vi "Close.vi"(8 "error in (no error)":errorcluster, 11 "QueueReader in":refnum<class "MultiQueueReader.lvclass">) -> (0 "error out":errorcluster, 3 "QueueReader out":refnum<class "MultiQueueReader.lvclass">)   [LabVIEW 2013, in "MultiQueueReader.lvclass"]
doc: "Closes all open references and reserved resources for the reader"
uses:
  MultiQueueReader.lvclass
  BaseReader/BaseReader.lvclass
  MultiQueueReader.lvclass/MultiQueueReader.ctl
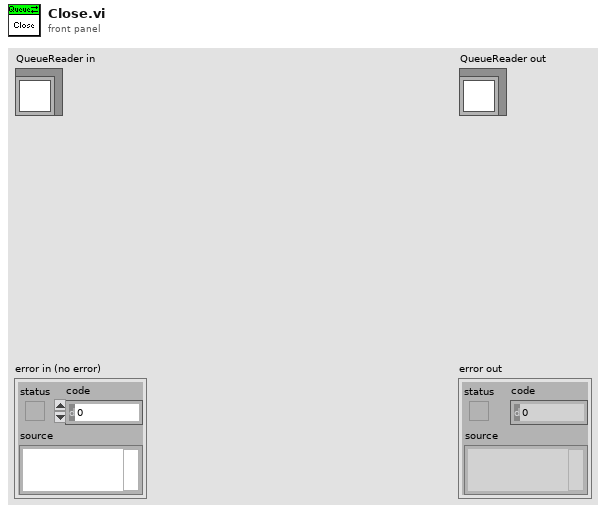
[diagram p1: front panel]
types:
  T1 = typedef "response queue.ctl" = refnum<queue>
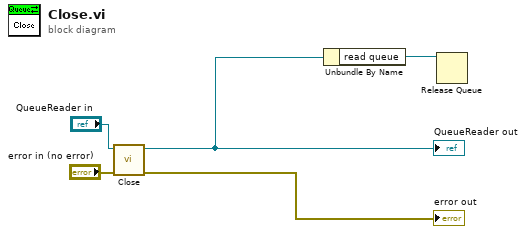
[diagram p0: block diagram]
diagram:
  n1 = call-parent "Close.vi"("error in (no error)"="error in (no error)", "BaseReader in"="QueueReader in") -> ("error out"=→"error out":errorcluster, "BaseReader out"=w1:refnum<class "MultiQueueReader.lvclass">)  [unwired: 8 in]
  "QueueReader out" <- w1
  n2 = Unbundle By Name(w1) -> ("read queue"=w2:T1)
  n3 = Release Queue(queue=w2) -> ()  [unwired: 2 in, 3 out]
